vi "Stop Core.vi"(10 "final error code":i32, 11 "Keepalive Heartbeat in":refnum<class "Keepalive Heartbeat.lvclass">) -> (3 "Keepalive Heartbeat out":refnum<class "Keepalive Heartbeat.lvclass">)   [LabVIEW 2021, in "WebSocket Actors.lvlib" / "Keepalive Heartbeat.lvclass"]
doc: "(<B>Filename</B>: Actor Framework.lvlib:Actor.lvclass:Stop Core.vi)\n\nDefines what the actor does before it stops. Use the <B>final error code</B> input to determine whether the actor shut down in response to an error.\n\nBy default, this method passes the Stop message along to all auto-stop nested actors. A descendant class may override this method to define additional behavior, such as shutting down any processes the actor initiated in its override of the Actor Core method."
uses:
  Keepalive Heartbeat.lvclass
  Keepalive Heartbeat.lvclass/Keepalive Heartbeat.ctl
  <vilib>/ActorFramework/Actor/Actor.lvclass
  <userlib>/_OpenG.lib/error/error.llb/openg_error.lvlib
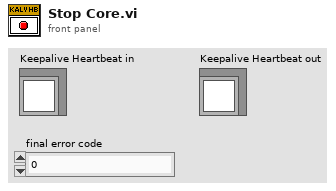
[diagram p1: front panel]
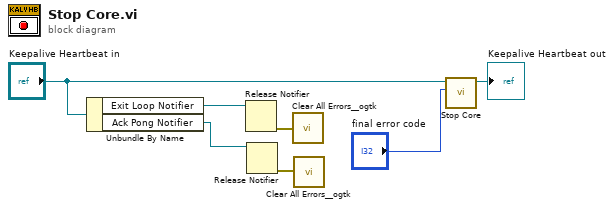
[diagram p0: block diagram]
diagram:
  n1 = Unbundle By Name("Keepalive Heartbeat in") -> ("Exit Loop Notifier"=w4:refnum<notifier>, "Ack Pong Notifier"=w3:refnum<notifier>)
  n2 = Release Notifier(notifier=w4) -> (error out=w2:errorcluster)  [unwired: 2 in, 2 out]
  n3 = Release Notifier(notifier=w3) -> (error out=w1:errorcluster)  [unwired: 2 in, 2 out]
  n4 = call <userlib>:"Clear All Errors__ogtk.vi"("Error In"=w2) -> ()  [unwired: 3 in, 1 out]
  n5 = call <userlib>:"Clear All Errors__ogtk.vi"("Error In"=w1) -> ()  [unwired: 3 in, 1 out]
  n6 = call-parent "Stop Core.vi"("final error code"="final error code", "Actor in"="Keepalive Heartbeat in") -> ("Actor out"=→"Keepalive Heartbeat out":refnum<class "Keepalive Heartbeat.lvclass">)  [unwired: 9 in]
